vi "Compass on new GIC D.vi"(11 "GIC Input":T1={"     Use ?\nOff       On"=[FALSE, TRUE, FALSE, TRUE], "Mode:"=FALSE, "Extra Port"="", "Hokuyo Port"="COM7", "Tx Prop  Port"="COM6", "Compass Port"="", "GPS Port"="", "Num of WPs"=0, "WP Lats and Longs"={"WP Lats"=[], "WP Longs"=[]}, "Obst Lats and Longs"={"Obst Lats"=[], "Obst Longs"=[]}, "Parameters"=[], "GPS Data"=[], "Compass"=0.0, "LMS Vector"=[], "Vision Vector"=[], "Direction Cmd"=0.0, "Speed Cmd"=0.0, "WP Vector"=[], "WP Number"=0, "Extra"=0, "SW Map"=[], "Path Cluster"={"Path x node"=[], "Path y node"=[]}, "Sim Course"=[]} {"Obst Lats and Longs"."Obst Longs" format="%#_8g"; "Obst Lats and Longs"."Obst Lats" format="%#_8g"}) -> (3 "GIC Output":T1={"     Use ?\nOff       On"=[FALSE, TRUE, FALSE, TRUE], "Mode:"=FALSE, "Extra Port"="", "Hokuyo Port"="COM7", "Tx Prop  Port"="COM6", "Compass Port"="", "GPS Port"="", "Num of WPs"=0, "WP Lats and Longs"={"WP Lats"=[], "WP Longs"=[]}, "Obst Lats and Longs"={"Obst Lats"=[], "Obst Longs"=[]}, "Parameters"=[], "GPS Data"=[], "Compass"=0.0, "LMS Vector"=[], "Vision Vector"=[], "Direction Cmd"=0.0, "Speed Cmd"=0.0, "WP Vector"=[], "WP Number"=0, "Extra"=0, "SW Map"=[], "Path Cluster"={"Path x node"=[], "Path y node"=[]}, "Sim Course"=[]} {"Obst Lats and Longs"."Obst Longs" format="%#_8g"; "Obst Lats and Longs"."Obst Lats" format="%#_8g"})   [LabVIEW 2014]
uses:
  Global_vars.vi
panel:
  out "compass out":dbl
  # "Compass on New GIC D - not working"
  # "Input:"
  # "Output:"
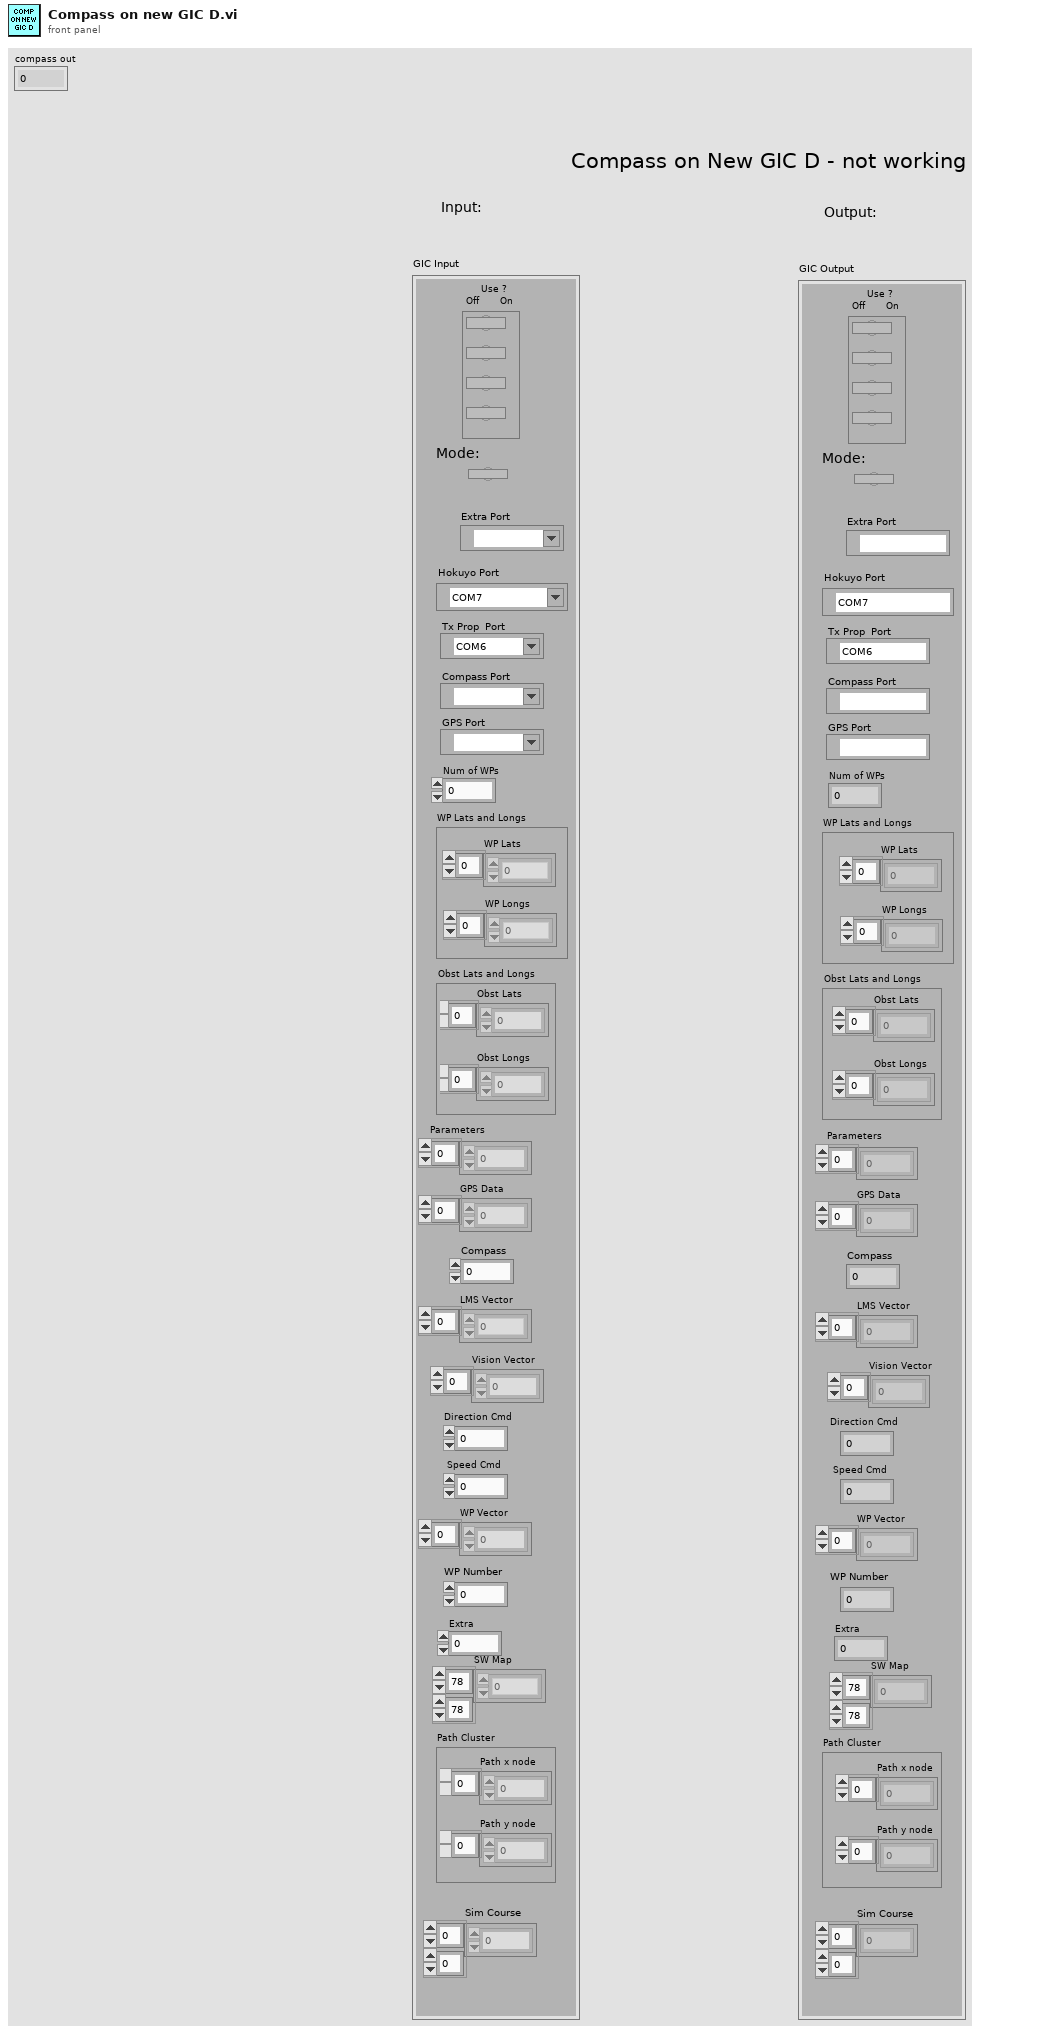
[diagram p1: front panel]
types:
  T1 = cluster{"     Use ?\nOff       On":bool[], "Mode:":bool, "Extra Port":refnum<visa-resource-name>, "Hokuyo Port":refnum<visa-resource-name>, "Tx Prop  Port":refnum<visa-resource-name>, "Compass Port":refnum<visa-resource-name>, "GPS Port":refnum<visa-resource-name>, "Num of WPs":i16, "WP Lats and Longs":cluster{"WP Lats":dbl[], "WP Longs":dbl[]}, "Obst Lats and Longs":cluster{"Obst Lats":dbl[], "Obst Longs":dbl[]}, "Parameters":dbl[], "GPS Data":dbl[], "Compass":dbl, "LMS Vector":dbl[], "Vision Vector":dbl[], "Direction Cmd":dbl, "Speed Cmd":dbl, "WP Vector":dbl[], "WP Number":i32, "Extra":i16, "SW Map":i32[][], "Path Cluster":cluster{"Path x node":dbl[], "Path y node":dbl[]}, "Sim Course":i8[][]}
  T2 = cluster{"     Use ?\nOff       On":bool[], "Mode:":bool, "Rx Prop Port":refnum<visa-resource-name>, "Hokuyo Port":refnum<visa-resource-name>, "Tx Prop  Port":refnum<visa-resource-name>, "Compass Port":refnum<visa-resource-name>, "GPS Port":refnum<visa-resource-name>, "Num of WPs":i16, "WP Lats and Longs":cluster{"WP Lats":dbl[], "WP Longs":dbl[]}, "Obst Lats and Longs":cluster{"Obst Lats":dbl[], "Obst Longs":dbl[]}, "Parameters":dbl[], "GPS Data":dbl[], "Compass":dbl, "LMS Vector":dbl[], "Vision Vector":dbl[], "Direction Cmd":dbl, "Speed Cmd":dbl, "WP Vector":dbl[], "WP Number":i32, "Extra":i16, "SW Map":i32[][], "Path Cluster":cluster{"Path x node":dbl[], "Path y node":dbl[]}, "Sim Course":i8[][]}
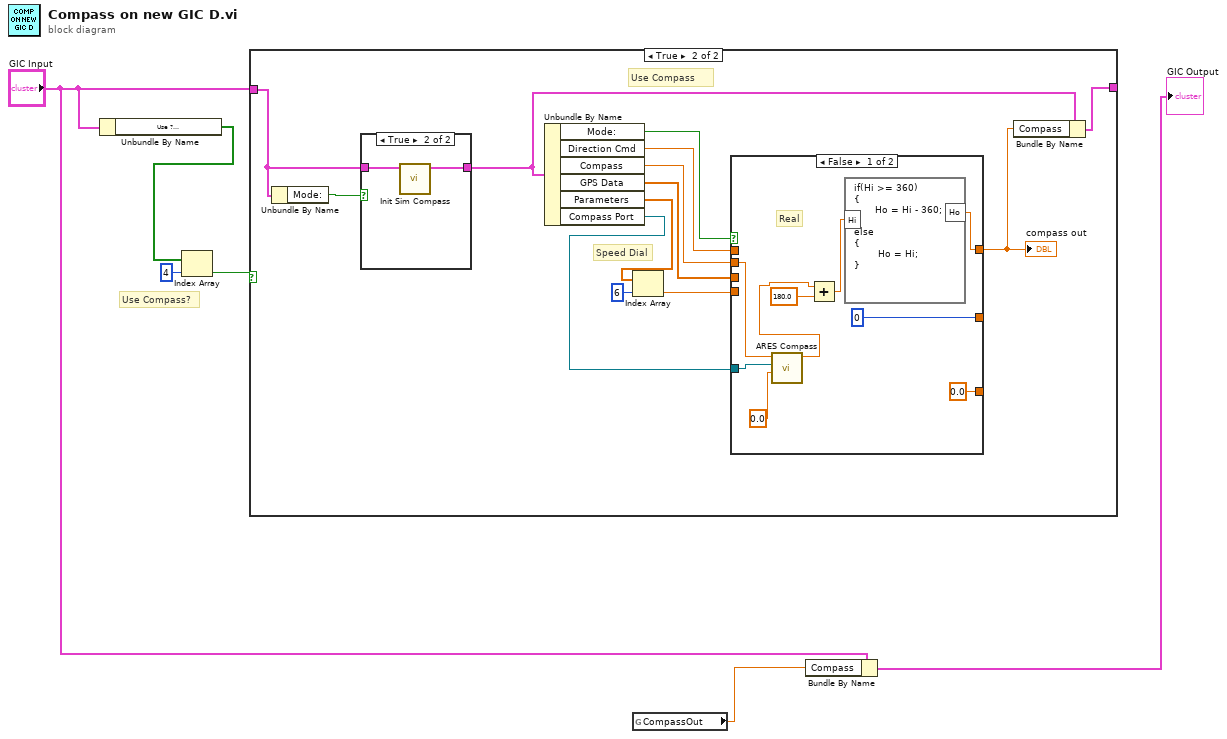
[diagram p0: block diagram]
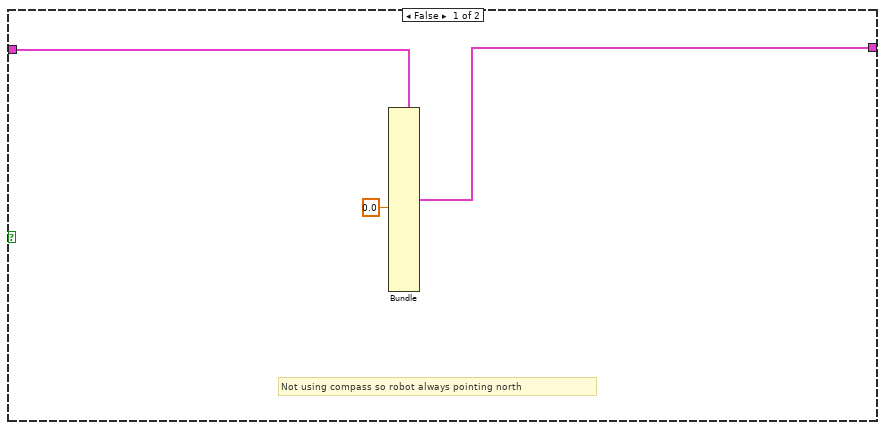
[diagram p2: hidden frame]
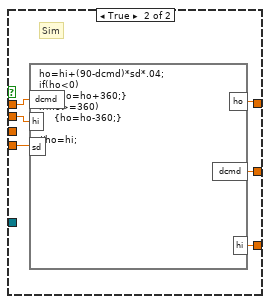
[diagram p4: hidden frame]
diagram:
  # "Use Compass?"
  n1 = Unbundle By Name("GIC Input") -> ("Use ?\nOff       On"=w6:bool[])
  n2 = Index Array(array=w6, index=4) -> (element=w4:bool)
  n3 = case shown="True" w4 {
    tunnel: "GIC Input" -> [w9 w11]
    tunnel: [w7 w17] -> _
    frame False {
      # "Not using compass so robot always pointing north"
      n4 = Bundle(cluster=w9, "Compass"=0.0) -> (w7:T1)  [unwired: 22 in]
    }
    frame True {
      # "Use Compass"
      # "Speed Dial"
      n5 = Unbundle By Name(w11) -> ("Mode:"=w12:bool)
      n6 = case shown="True" w12 {
        tunnel: w11 -> [w23 w25]
        tunnel: [w23 w24] -> w10
        frame False {
        }
        frame True {
          n7 = call "Init Sim Compass.vi"("GIC Input"=w25) -> ("GIC Output"=w24:T2)  [unwired: 10 in]
        }
      }
      n8 = Unbundle By Name(w10) -> ("Mode:"=w21:bool, "Direction Cmd"=w16:dbl, "Compass"=w15:dbl, "GPS Data"=w22:dbl[], "Parameters"=w20:dbl[], "Compass Port"=w13:refnum<visa-resource-name>)
      n9 = Index Array(array=w20, index=6) -> (element=w18:dbl)
      n10 = case shown="False" w21 {
        tunnel: w16 -> [_ w39]
        tunnel: w15 -> [w32 w38]
        tunnel: [w27 w40] -> w14
        tunnel: w22 -> [_ _]
        tunnel: w18 -> [_ w37]
        tunnel: [0 w36] -> _
        tunnel: [0.0 ("hi") w35] -> _
        tunnel: w13 -> [w31 _]
        frame False {
          # "Real"
          n11 = call "ARES Compass.vi"("Input time of last compass read"=0.0, "Compass Com Port"=w31, "Compass In"=w32) -> ("Compass Out"=w28:dbl)  [unwired: 6 in, 1 out]
          n12 = Add(x=w28, y=180.0) -> (x+y=w26:dbl)
          n13 = formula code="if(Hi >= 360)\n{\n       Ho = Hi - 360;\n}\nelse\n{\n        Ho = Hi;\n}"("Hi"=w26) -> ("Ho"=w27:dbl)
        }
        frame True {
          # "Sim"
          n14 = formula code="ho=hi+(90-dcmd)*sd*.04;\nif(ho<0)\n     {ho=ho+360;}\nif(ho>=360)\n     {ho=ho-360;}\n\n//ho=hi;"("dcmd"=w39, "hi"=w38, "sd"=w37) -> ("ho"=w40:dbl, "dcmd"=w36:dbl, "hi"=w35:dbl)
        }
      }
      "compass out" <- w14
      n15 = Bundle By Name(cluster=w10, "Compass"=w14) -> (w17:T2)
    }
  }
  n16 = global read "Global_vars.vi" "CompassOut"() -> (w2:dbl)
  n17 = Bundle By Name(cluster="GIC Input", "Compass"=w2) -> (→"GIC Output":T1)
